vi "SQLite Backup Old TestSequenceItems.vi"(8 "error in (no error)":errorcluster, 10 "Items":string="0", 11 "Main":string="0") -> (0 "error out":errorcluster)   [LabVIEW 2017, in "SQLite.lvclass"]
doc: "保存校准的结果值,.\n2015-11-03 16:29:50\nBy：蒋松\nEmail：jiangsong@outlook.com\nSina: @sushu1051"
uses:
  SQLite.lvclass
  SQLiteFileName.ctl
  TabelFullName.ctl
  <vilib>/Utility/error.llb/Trim Whitespace.vi
  <userlib>/LabSQL/LabSQL.lvlib
  <userlib>/sushu/sushu.lvlib
panel:
  out "Numeric":i32
  in  "SequenceNum":string
  out "Result Set":string[][](table) caption="Result Set (from first statement with results)"
  # "insert 之前要先删除所有的就的校准值。\n2015-11-03 16:45:40\nBy：蒋松\nEmail：jiangsong@outlook.com\nSina: @sushu1051"
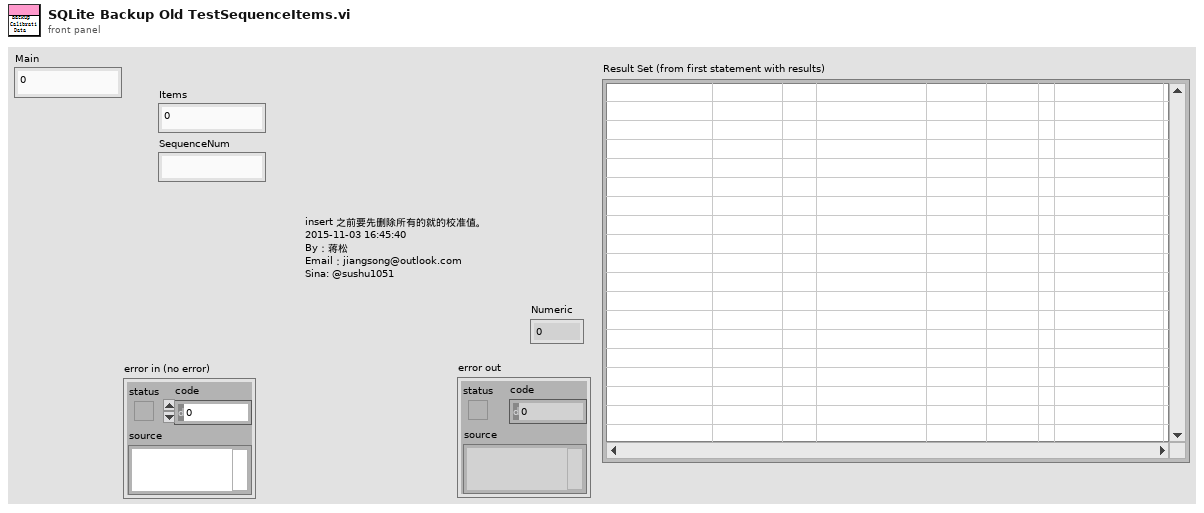
[diagram p1: front panel]
types:
  T1 = typedef "SQLite.lvclass/TabelFullName.ctl" = string
  T2 = typedef "SQLite.lvclass/SQLiteFileName.ctl" = string
  T3 = enum32{"invalid app kind", "Development System", "Run Time System", "Student Edition", "Embedded LabVIEW", "Evaluation", "Custom"}
  T4 = enum32{"Invalid", "Standard", "Closed", "Hidden", "Minimized", "Maximized"}
  T5 = enum16{"Other", "SQL2008", "SQLite", "Access", "MySQL"}
  T6 = cluster{"Core":cluster{"Current VI Reference":refnum<vi>, "Close Panel on Exit?":bool}}
  T7 = cluster{"Current VI Reference":refnum<vi>, "Close Panel on Exit?":bool}
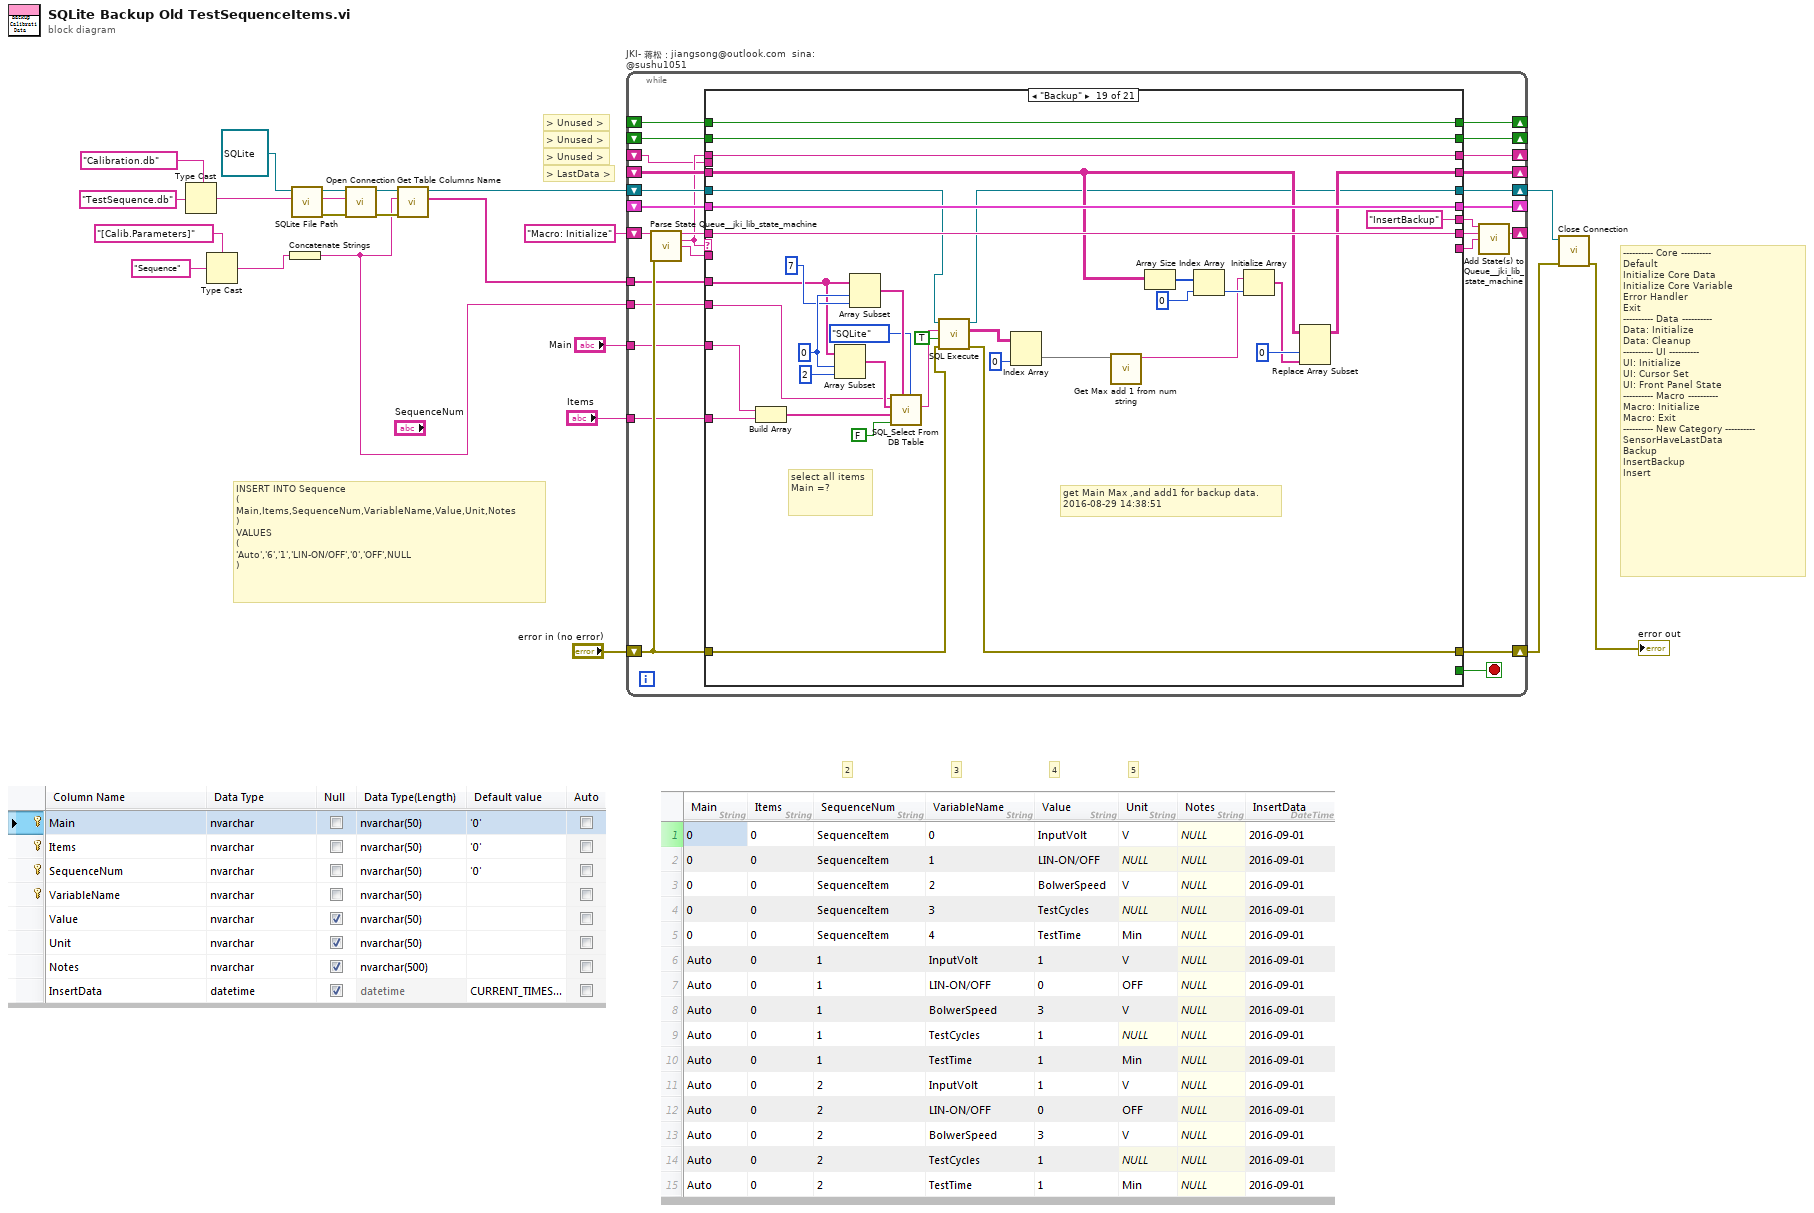
[diagram p0: block diagram]
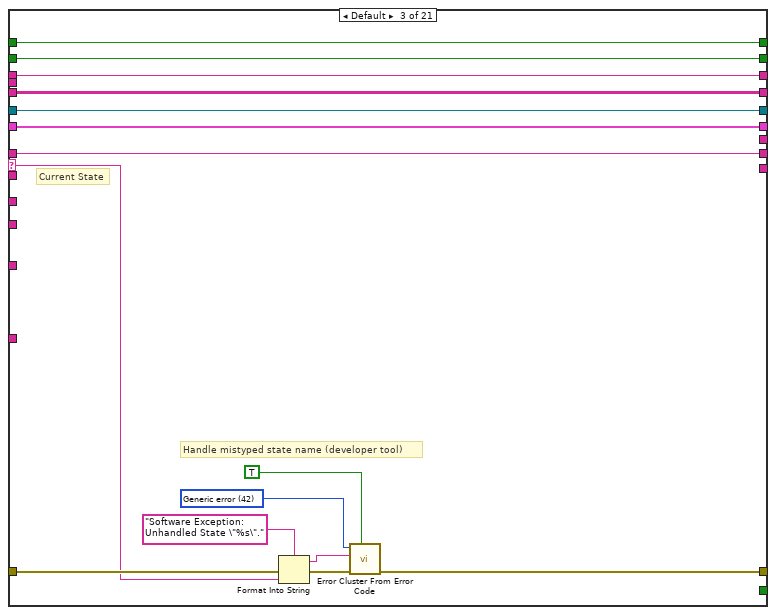
[diagram p4: hidden frame]
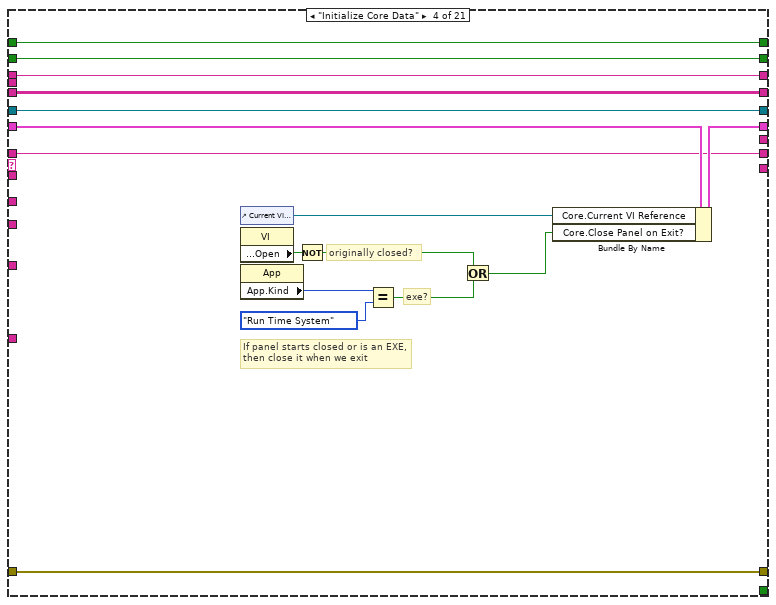
[diagram p5: hidden frame]
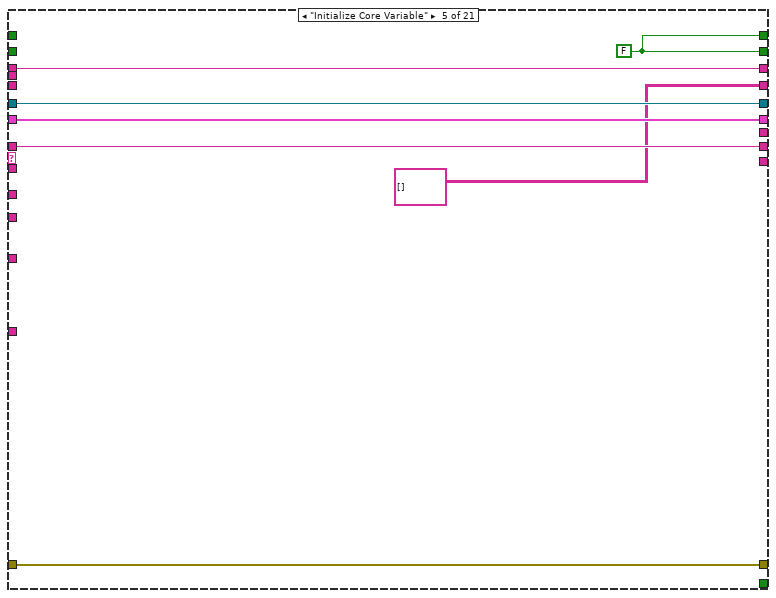
[diagram p6: hidden frame]
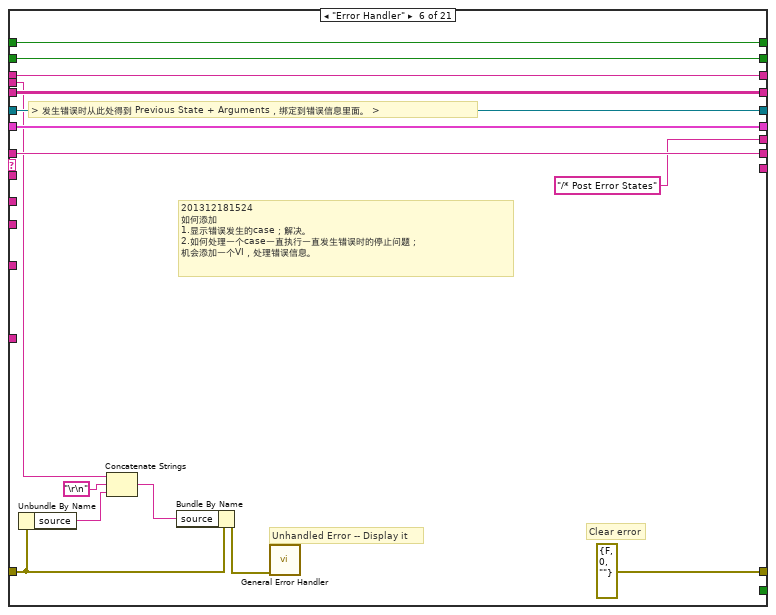
[diagram p7: hidden frame]
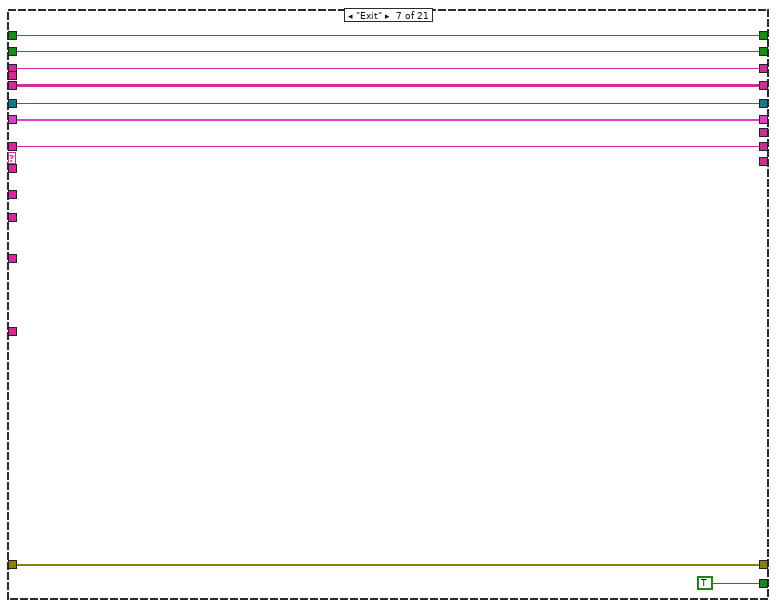
[diagram p8: hidden frame]
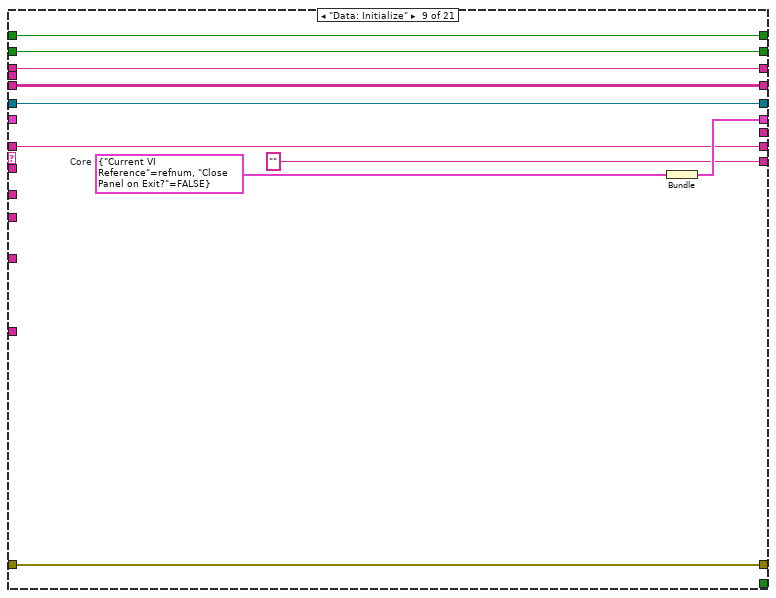
[diagram p10: hidden frame]
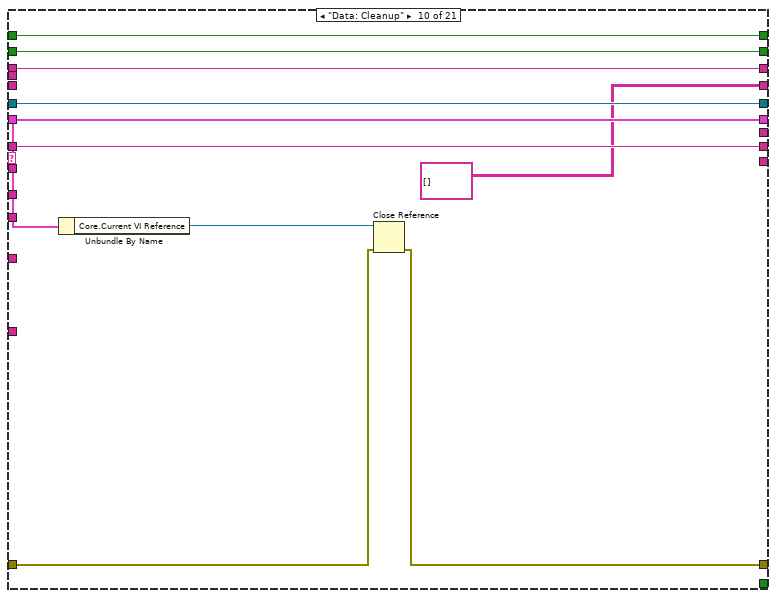
[diagram p11: hidden frame]
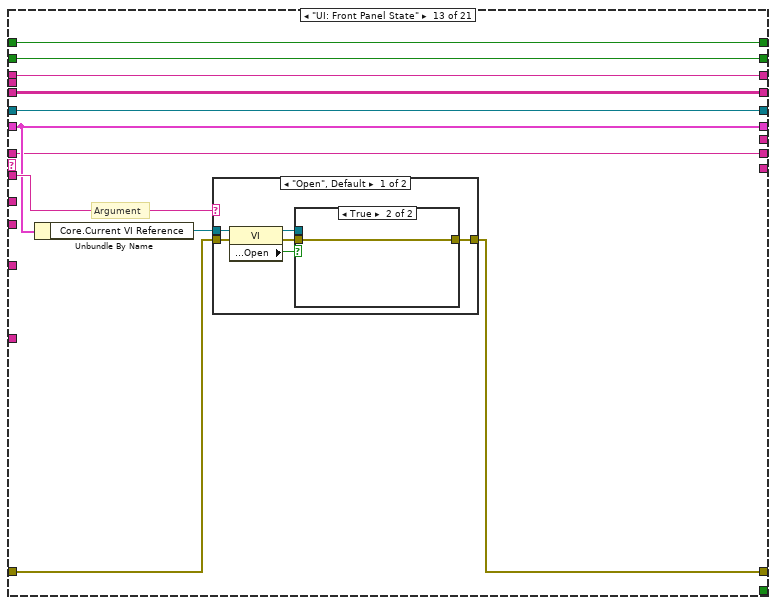
[diagram p14: hidden frame]
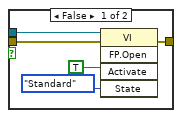
[diagram p15: hidden frame]
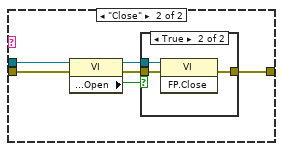
[diagram p16: hidden frame]
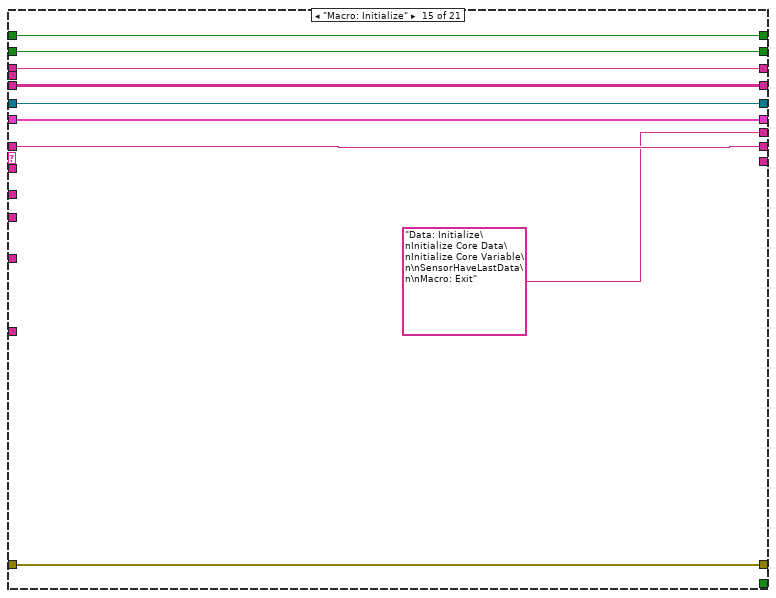
[diagram p19: hidden frame]
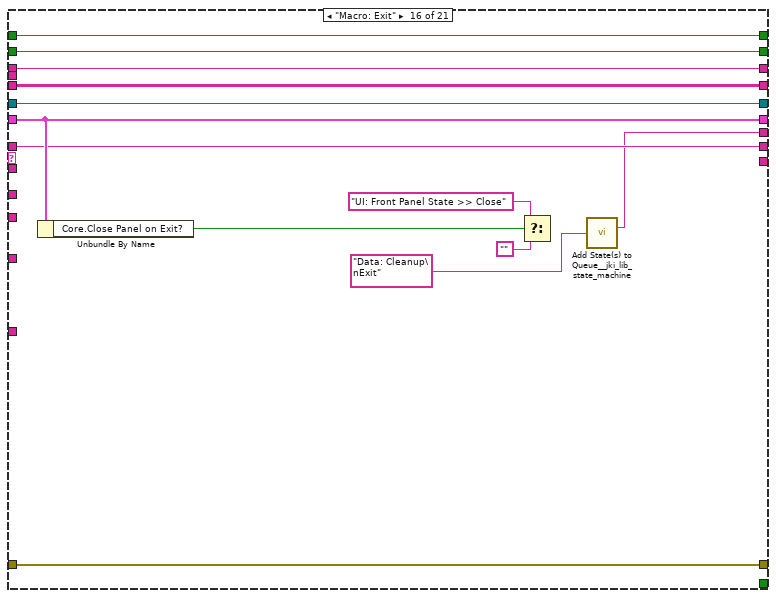
[diagram p20: hidden frame]
diagram:
  # "INSERT INTO Sequence\n(\nMain,Items,SequenceNum,VariableName,Value,Unit,Notes\n)\nVALUES\n(\n'Auto','6','1','LIN-ON/OFF','0','OFF',NULL\n)"
  # "5"
  # "4"
  # "3"
  # "2"
  # "> Unused >"
  # "> LastData >"
  # "> Unused >"
  # "> Unused >"
  # "---------- Core ----------\nDefault\nInitialize Core Data\nInitialize Core Variable\nError Handler\nExit\n---------- Data ----------\nData: Initialize\nData: Cleanup\n---------- UI ----------\nUI: Initialize\nUI: Cursor Set\nUI: Front Panel State\n---------- Macro ----------\nMacro: Initialize\nMacro: Exit\n---------- New Category ----------\nSensorHaveLastData\nBackup\nInsertBackup\nInsert"
  n1 = Type Cast(type=T2 "Calibration.db" ("SQLiteFileName"), x="TestSequence.db" ("Remaining States")) -> (*(type *) &x=w10:T2)
  n2 = Type Cast(type=T1 "[Calib.Parameters]" ("TabelFullName"), x="Sequence" ("Remaining States")) -> (*(type *) &x=w7:T1)
  n3 = Concatenate Strings(w7) -> (w4:string)
  n4 = call "SQLite File Path.vi"("SQLiteFileName"=w10, "SQLite in"=refnum<class "SQLite.lvclass"> refnum ("SQLite.lvclass")) -> ("error out"=w13:errorcluster, "string"=w16:string, "SQLite out"=w14:refnum<class "SQLite.lvclass">)  [unwired: 7 in]
  n5 = call-dynamic "Open Connection.vi"("error in (no error)"=w13, "ConnectionString"=w16, "HostDB in"=w14) -> ("error out"=w17:errorcluster, "HostDB out"=w18:refnum<class "SQLite.lvclass">)  [unwired: 7 in]
  n6 = call-dynamic "Get Table Columns Name.vi"("error in (no error)"=w17, "TableName"=w4, "HostDB in"=w18) -> ("ColunmsList"=w6:string[], "HostDB out"=w5:refnum<class "SQLite.lvclass">)  [unwired: 4 in, 3 out]
  n7 = while "JKI- 蒋松：jiangsong@outlook.com  sina: @sushu1051" {
    shift-right: [w47] -> w2
    shift-left: "error in (no error)" -> [w45]
    shift-right: [w35] -> _
    shift-left: "Macro: Initialize" -> [w36]
    shift-right: [w42] -> _
    shift-left: _ -> [w23]
    shift-right: [w43] -> _
    shift-left: _ -> [w44]
    shift-right: [w37] -> _
    shift-left: _ -> [w40]
    shift-right: [w38] -> w3
    shift-left: w5 -> [w31]
    shift-right: [w39] -> _
    shift-left: _ -> [w41]
    shift-right: [w30] -> _
    shift-left: _ -> [w29]
    tunnel: w6 -> [w28]
    tunnel: w4 -> [w27]
    tunnel: "Main" -> [w26]
    tunnel: "Items" -> [w25]
    stop <- w46 stop-if-true
    n8 = call <vilib>:"Parse State Queue__jki_lib_state_machine.vi"("State Queue"=w36, "Error In (no error)"=w45) -> ("Remaining States"=w49:string, "Current State"=w24:string, "Arguments"=w48:string)  [unwired: 10 in, 1 out]
    n9 = case shown="\"Backup\"" w24 {
      selector: w24 -> [_ _ w68 _ _ _ _ _ _ _ _ _ _ _ _ _ _ _ _ _ _]
      tunnel: w49 -> [w57 w59 w67 w82 w101 w108 w120 w129 w138 w148 w157 w165 w173 w206 w215 w224 w236 w267 w302 w327 w346]
      tunnel: w48 -> [_ _ _ _ _ _ _ _ _ _ _ _ w176 _ _ _ _ _ _ _ _]
      tunnel: [w56 w65 w69 w93 w103 errorcluster {"status"=FALSE, "code"=0, "source"=""} ("error out") w122 w131 w142 w150 w159 w167 w177 w208 w217 w231 w239 w245 w273 w308 w347] -> w47
      tunnel: w45 -> [w56 w65 w70 w93 w103 w112 w122 w131 w142 w151 w159 w167 w178 w208 w217 w231 w239 w246 w274 w320 w347]
      tunnel: [w57 w59 w67 w82 w101 w108 w120 w129 w138 w148 w157 w165 w173 w206 w215 w224 w236 w267 w302 w327 w346] -> w34
      tunnel: [_ _ _ _ _ _ TRUE _ _ _ _ _ _ _ _ _ _ _ _ _ _] -> w46
      tunnel: w44 -> [w55 w64 w80 w96 _ w118 w127 w135 w145 w155 w163 w171 w182 w212 w221 w234 w242 w270 w305 w326 w345]
      tunnel: w24 -> [w54 w63 w79 w95 w97 w117 w126 w134 w144 w154 w162 w170 w181 w211 w220 w233 w241 w269 w304 w325 w344]
      tunnel: [w55 w64 w80 w96 w100 w118 w127 w135 w145 w155 w163 w171 w182 w212 w221 w234 w242 w270 w305 w326 w345] -> w43
      tunnel: [w54 w63 w79 w95 w97 w117 w126 w134 w144 w154 w162 w170 w181 w211 w220 w233 w241 w269 w304 w325 w344] -> w42
      tunnel: w41 -> [w53 w62 w78 w94 _ w116 w125 w133 w143 _ w161 w169 w180 w210 w219 w232 w240 _ w283 w313 w343]
      tunnel: w31 -> [w51 w60 w77 w83 w99 w106 w121 w130 w139 w149 w158 w166 w174 w207 w216 w225 w237 w250 w276 w322 w342]
      tunnel: w40 -> [w52 w61 w76 w85 w102 w115 w124 w132 _ w152 w160 w168 w175 w209 w218 w226 w238 w268 w303 w324 w341]
      tunnel: [w53 w62 w78 w94 string[][] [] ("Result Set") w116 w125 w133 w143 string[][] [] ("Result Set") w161 w169 w180 w210 w219 w232 w240 w248 w293 w313 w343] -> w39
      tunnel: [w51 w60 w77 w83 w99 w106 w121 w130 w139 w149 w158 w166 w174 w207 w216 w225 w237 w249 w277 w321 w342] -> w38
      tunnel: [w52 w61 w76 w84 w102 w115 w124 w132 w140 w152 w160 w168 w175 w209 w218 w226 w238 w268 w303 w324 w341] -> w37
      tunnel: [_ _ _ _ _ "/* Post Error States" _ _ _ _ _ _ _ _ "Data: Initialize\nInitialize Core Data\nInitialize Core Variable\n\nSensorHaveLastData\n\nMacro: Exit" w223 _ w257 "InsertBackup" ("Remaining States") _ _] -> w33
      tunnel: [_ _ _ _ _ _ _ _ "" _ _ _ _ _ _ _ _ _ _ _ _] -> w32
      tunnel: w29 -> [w50 w58 w66 w81 _ w105 w119 w128 w136 w147 w156 w164 w172 w205 w213 w222 w235 w266 w301 w323 w340]
      tunnel: [w50 w58 w66 w81 w100 w105 w119 w128 w136 w147 w156 w164 w172 w205 w213 w222 w235 w266 w301 w323 w340] -> w30
      tunnel: w28 -> [_ _ _ _ _ _ _ _ _ _ _ _ _ _ _ _ _ w256 w286 w319 _]
      tunnel: w27 -> [_ _ _ _ _ _ _ _ _ _ _ _ _ _ _ _ _ w263 w285 w314 _]
      tunnel: w26 -> [_ _ _ _ _ _ _ _ _ _ _ _ _ _ _ _ _ w261 w284 w312 _]
      tunnel: w25 -> [_ _ _ _ _ _ _ _ _ _ _ _ _ _ _ _ _ w252 w280 w311 _]
      tunnel: w23 -> [_ _ _ _ _ w104 _ _ _ _ _ _ _ _ _ _ _ _ _ _ _]
      frame "Idle" {
      }
      frame "---------- Core ----------" {
      }
      frame Default {
        w72 = 42 items=["No error", "Argument error", "Memory is full", "Out of zone", "End of file", "File already open", "Generic file I/O error", "File not found", "File permission error", "Disk is full", "Duplicate path", "Too many files open", "System feature not enabled", "Resource file not found", "Cannot add resource", "Resource not found", "Image not found", "Image memory error", "Pen does not exist", "Config type invalid", "Config token not found", "Config parse error", "Config memory error", "Bad external code format", "Bad external code offset", "External code not present", "Null window", "Destroy window error", "Null menu", "Print aborted", "Bad print record", "Print driver error", "Windows error during printing", "Memory error during printing", "Print dialog error", "Generic print error", "Invalid device refnum", "Device not found", "Device parameter error", "Device unit error", "Cannot open device", "Device call aborted", "Generic error", "Cancelled by user", "Object ID too low", "Object ID too high", "Object not in heap", "Unknown heap", "Unknown object (invalid DefProc)", "Unknown object (DefProc not in table)", "Message out of range", "Invalid (null) method", "Unknown message", "Manager call not supported", "Bad address", "Network operation in progress", "Network operation timed out", "Connection is busy", "Network attribute not supported", "Network error", "Address in use", "System out of memory", "Connection aborted", "Connection refused", "Not connected", "Already connected", "Connection closed", "Initialization error (interapplication manager)", "Bad occurrence", "Wait on unbound occurrence handler", "Occurrence queue overflow", "Datalog type conflict", "Unused", "Unrecognized type (interapplication manager)", "Memory corrupt", "Failed to make temporary DLL", "Old CIN version", "Drag socket not found", "Failed to load drop-object", "Failed to register OLE object", "Failed to release OLE object", "Format specifier type mismatch", "Unknown format specifier", "Too few format specifiers", "Too many format specifiers", "Scan failed", "Newer CIN version", "Error converting to variant", "Runtime menu error", "Password tampered", "Variant attribute not found", "Incompatible variant data type", "Event data is not available", "Event Store is not present", "Occurrence is not found", "Event Queue is not created", "Event info is not available", "Refnum passed is NULL", "Error retrieving Class GUID", "Error retrieving CoClass GUID", "Error retrieving TypeLib GUID.", "Bad built application magic bytes.", "Specific driver is different from the specific driver associated with the Logical Name.", "There is no session opened to the class driver.", "Max Error", "MAX - Error with config objects", "MAX - Error loading configuration", "MAX - Group not supported"]
        # "Current State"
        # "Handle mistyped state name (developer tool)"
        n10 = Format Into String(format string="Software Exception: Unhandled State \"%s\"." ("message"), error in=w70, w68) -> (resulting string=w73:string, error out=w74:errorcluster)  [unwired: 1 in]
        n11 = call <vilib>:"Error Cluster From Error Code.vi"("show call chain? (False)"=TRUE, "error in (no error)"=w74, "error message (\"\")"=w73, "error code (0)"=w72) -> ("error out"=w69:errorcluster)  [unwired: 5 in]
      }
      frame "Initialize Core Data" {
        # "originally closed?"
        # "exe?"
        # "If panel starts closed or is an EXE, then close it when we exit"
        n12 = control-ref of="Current VI Reference"() -> (w92:refnum<vi>)
        n13 = property class="VI"() -> ("Front Panel.Open"=w86:bool)  [unwired: 2 in, 2 out]
        n14 = property class="App"() -> ("App.Kind"=w87:T3)  [unwired: 2 in, 2 out]
        n15 = Not(x=w86) -> (.not. x?=w89:bool)
        n16 = Equal?(x=w87, y=T3."Run Time System" ("Application:Kind")) -> (x = y?=w90:bool)
        n17 = Or(x=w89, y=w90) -> (x .or. y?=w91:bool)
        n18 = Bundle By Name(cluster=w85, "Core.Current VI Reference"=w92, "Core.Close Panel on Exit?"=w91) -> (w84:T6)
      }
      frame "Initialize Core Variable" {
        w100 = FALSE
      }
      frame "Error Handler" {
        # "> 发生错误时从此处得到 Previous State + Arguments，绑定到错误信息里面。 >"
        # "201312181524\n如何添加\n1.显示错误发生的case；解决。\n2.如何处理一个case一直执行一直发生错误时的停止问题；\n机会添加一个VI，处理错误信息。"
        # "Clear error"
        # "Unhandled Error -- Display it"
        n19 = Unbundle By Name(w112) -> ("source"=w110:string)
        n20 = Concatenate Strings(w104, "\r\n", w110) -> (w109:string)
        n21 = Bundle By Name(cluster=w112, "source"=w109) -> (w113:errorcluster)
        n22 = call <vilib>:"General Error Handler.vi"("error in (no error)"=w113) -> ()  [unwired: 10 in, 5 out]
      }
      frame "Exit" {
      }
      frame "---------- Data ----------" {
      }
      frame "Data: Initialize" {
        w141 = T7 {"Current VI Reference"=refnum, "Close Panel on Exit?"=FALSE}  # Core
        n23 = Bundle("Core"=w141) -> (w140:T6)  [unwired: 1 in]
      }
      frame "Data: Cleanup" {
        n24 = Unbundle By Name(w152) -> ("Core.Current VI Reference"=w153:refnum<vi>)
        n25 = Close Reference(reference=w153, error in (no error)=w151) -> (error out=w150:errorcluster)
      }
      frame "---------- UI ----------" {
      }
      frame "UI: Initialize" {
      }
      frame "UI: Front Panel State" {
        # "Argument"
        n26 = Unbundle By Name(w175) -> ("Core.Current VI Reference"=w179:refnum<vi>)
        n27 = case shown="\"Open\", Default" w176 {
          tunnel: w178 -> [w186 w199]
          tunnel: [w188 w200] -> w177
          tunnel: w179 -> [w187 w197]
          frame "Open", Default {
            n28 = property class="VI"(reference=w187, error in=w186) -> (reference out=w184:refnum<vi>, error out=w185:errorcluster, "Front Panel.Open"=w183:bool)
            n29 = case shown="True" w183 {
              tunnel: [w191 w194] -> w188
              tunnel: w185 -> [w190 w194]
              tunnel: w184 -> [w189 _]
              frame False {
                n30 = invoke class="VI" method="FP.Open"(reference=w189, error in=w190, "Activate"=TRUE, "State"=T4."Standard") -> (error out=w191:errorcluster)  [unwired: 1 in, 4 out]
              }
              frame True {
              }
            }
          }
          frame "Close" {
            n31 = property class="VI"(reference=w197, error in=w199) -> (reference out=w196:refnum<vi>, error out=w198:errorcluster, "Front Panel.Open"=w195:bool)
            n32 = case shown="True" w195 {
              tunnel: [w201 w204] -> w200
              tunnel: w198 -> [w201 w203]
              tunnel: w196 -> [_ w202]
              frame False {
              }
              frame True {
                n33 = invoke class="VI" method="FP.Close"(reference=w202, error in=w203) -> (error out=w204:errorcluster)  [unwired: 1 in, 2 out]
              }
            }
          }
        }
      }
      frame "---------- Macro ----------" {
      }
      frame "Macro: Initialize" {
      }
      frame "Macro: Exit" {
        n34 = Unbundle By Name(w226) -> ("Core.Close Panel on Exit?"=w227:bool)
        n35 = Select(t="UI: Front Panel State >> Close", s=w227, f="") -> ()  [unwired: 1 out]
        n36 = call <vilib>:"Add State(s) to Queue__jki_lib_state_machine.vi"("State(s) at Back (\"\")"="Data: Cleanup\nExit") -> ("States Out"=w223:string)  [unwired: 14 in]
      }
      frame "---------- New Category ----------" {
      }
      frame "SensorHaveLastData" {
        w255 = 0 ("index")
        n37 = Build Array(w261, w252) -> (w262:string[])
        n38 = Array Subset(array=w256, index=w255, length=2) -> (w265:string[])
        n39 = Array Subset(array=w256, index=w255, length=7) -> (w253:string[])
        n40 = call <userlib>:"SQL_Select From DB Table.vi"("DB Type"=T5."SQLite", "SelectedColumnsNameList"=w253, "Check ASCII?"=FALSE, "ColumnsValue"=w262, "ColumnsNameList"=w265, "TableName"=w263) -> ("Select SQL CMD"=w247:string)  [unwired: 5 in]
        n41 = call-dynamic "SQL Execute.vi"("error in (no error)"=w246, "Return Data (T)"=TRUE, "Command Text"=w247, "HostDB in"=w250) -> ("error out"=w245:errorcluster, "Table Control"=w248:string[][], "HostDB out"=w249:refnum<class "SQLite.lvclass">)  [unwired: 3 in, 2 out]
        "Result Set" <- w248
        n42 = Empty Array?(array=w248) -> (empty?=w260:bool)
        n43 = Select(t="Insert" ("Remaining States"), s=w260, f="Backup" ("Remaining States")) -> (s? t:f=w257:string)
      }
      frame "Backup" {
        w289 = 0 ("index")
        # "select all items \nMain =?"
        # "get Main Max ,and add1 for backup data.\n2016-08-29 14:38:51"
        n44 = Build Array(w284, w280) -> (w290:string[])
        n45 = Array Subset(array=w286, index=w289, length=2) -> (w292:string[])
        n46 = Array Subset(array=w286, index=w289, length=7) -> (w287:string[])
        n47 = call <userlib>:"SQL_Select From DB Table.vi"("DB Type"=T5."SQLite", "SelectedColumnsNameList"=w287, "Check ASCII?"=FALSE, "ColumnsValue"=w290, "ColumnsNameList"=w292, "TableName"=w285) -> ("Select SQL CMD"=w275:string)  [unwired: 5 in]
        n48 = call-dynamic "SQL Execute.vi"("error in (no error)"=w274, "Return Data (T)"=TRUE, "Command Text"=w275, "HostDB in"=w276) -> ("error out"=w273:errorcluster, "Table Control"=w278:string[][], "HostDB out"=w277:refnum<class "SQLite.lvclass">)  [unwired: 3 in, 2 out]
        n49 = Index Array(array=w278, index (col)=0 ("disabled index (col)")) -> (element=w282:string[])  [unwired: 1 in]
        n50 = call <userlib>:"Get Max add 1 from num string.vi"("Input Array"=w282) -> ("Max Num +1"=w281:string)  [unwired: 9 in, 1 out]
        n51 = Array Size(array=w283) -> (size(s)=w298:i32[])
        n52 = Index Array(array=w298, index=0) -> (element=w296:i32)
        n53 = Initialize Array(w281, w296) -> (w295:string[])
        n54 = Replace Array Subset(array=w283, new element=w295, index (col)=0 ("disabled index (col)")) -> (w293:string[][])  [unwired: 1 in]
      }
      frame "InsertBackup" {
        w316 = 7 ("length")
        w317 = 0 ("index")
        n55 = Array Subset(array=w319, index=w317, length=w316) -> (w318:string[])
        n56 = Array Subset(array=w313, index (col)=w317, length (col)=w316) -> (w315:string[][])  [unwired: 2 in]
        n57 = for {
          tunnel: w314 -> [w339]
          tunnel: w318 -> [w338]
          shift-right: [w332] -> w321
          shift-left: w322 -> [w333]
          tunnel: w315 -> [w337] mode=indexing
          tunnel: w320 -> [w331]
          tunnel: [w330] -> w309
          tunnel: FALSE ("Return Data (T)") -> [w329]
          tunnel: enum16{"Other", "SQL2008", "SQLite"}."SQLite" ("DB Type") -> [w328]
          i -> [w335]
          n58 = call <userlib>:"SQL_Insert DB Table.vi"("DB Type"=w328, "ColumnsValue"=w337, "ColumnsName"=w338, "Table Name"=w339) -> ("Insert DB String"=w334:string)  [unwired: 7 in]
          n59 = call-dynamic "SQL Execute.vi"("error in (no error)"=w331, "Return Data (T)"=w329, "Command Text"=w334, "HostDB in"=w333) -> ("error out"=w330:errorcluster, "HostDB out"=w332:refnum<class "SQLite.lvclass">)  [unwired: 3 in, 3 out]
          n60 = Wait Until Next ms Multiple(millisecond multiple=u32 2) -> ()  [unwired: 1 out]
          "Numeric" <- w335
        }
        n61 = call <vilib>:"Add State(s) to Queue__jki_lib_state_machine.vi"("State(s) in (\"\")"=w312, "State(s) at Back (\"\")"=w311) -> ("States Out"=w310:string)  [unwired: 13 in]
        n62 = call "SQLite Delete Items of TestSequence.vi"("error in (no error)"=w309, "Main"=w310) -> ("error out"=w308:errorcluster)  [unwired: 8 in, 1 out]
      }
      frame "Insert" {
      }
    }
    n63 = call <vilib>:"Add State(s) to Queue__jki_lib_state_machine.vi"("State(s) in Front (\"\")"=w33, "State(s) in (\"\")"=w34, "State(s) at Back (\"\")"=w32) -> ("States Out"=w35:string)  [unwired: 12 in]
  }
  n64 = call-dynamic "Close Connection.vi"("error in (no error)"=w2, "HostDB in"=w3) -> ("error out"=→"error out":errorcluster)  [unwired: 8 in, 1 out]
